vi "FRCts20_Backend_RequestRoot_POST.vi"(6 "Message Attributes":T4, 8 "error in (no error)":errorcluster, 10 "Data":string, 11 "Engine_Refnums":T1) -> (0 "error out":errorcluster)   [LabVIEW 2013, in "FRCts20_Backend_Engine.lvlib"]
doc: "Adds a new request, called by the Request Root API. Expects the team index and description, returns the new request's index"
uses:
  FRCts20_Backend_Engine.lvlib
  Dependencies/Keyed Array/KeyedArray.ctl
  FRCts20_Backend_EngineRefnums.ctl
  INI_Accessor/FRCts20_Backend_INI Controller.lvclass
  Dependencies/AMC/_SubVIs/TypeDefs/Message Queue.ctl
  Dependencies/AMC/_SubVIs/TypeDefs/Message.ctl
  <vilib>/addons/database/Connection.llb/Conn ObjectReference.ctl
  FRCts20_Backend_FGVOperation.ctl
  FRCts20_Backend_API/FRCts20_Backend_API_RequestRoot.ctl
  FRCts20_Backend_API/FRCts20_Backend_API_Status.ctl
  FRCts20_Backend_API/FRCts20_Backend_API.lvlib
  Dependencies/Keyed Array/Tools_KeyedArray.lvlib
  Dependencies/AMC/AMC.lvlib
  <vilib>/addons/database/NI_Database_API.lvlib
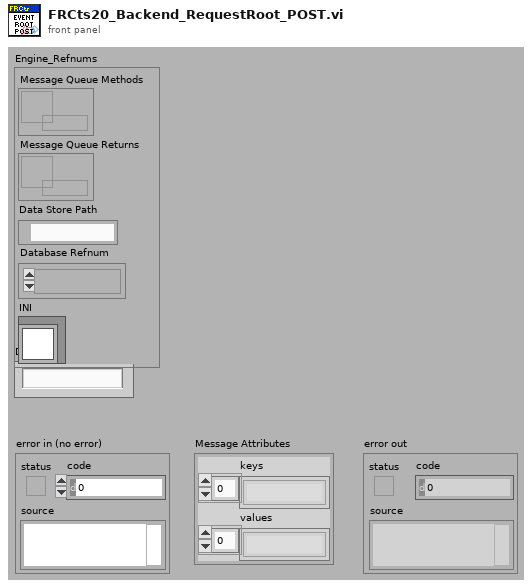
[diagram p1: front panel]
types:
  T1 = typedef "FRCts20_Backend_Engine.lvlib/FRCts20_Backend_EngineRefnums.ctl" = cluster{"Message Queue Methods":T2, "Message Queue Returns":T2, "Data Store Path":path, "Database Refnum":T3, "INI":refnum<class "FRCts20_Backend_INI Controller.lvclass">}
  T2 = typedef "AMC.lvlib/Message Queue.ctl" = refnum<queue>
  T3 = typedef "NI_Database_API.lvlib/Conn ObjectReference.ctl" = refnum<k1>
  T4 = typedef "Tools_KeyedArray.lvlib/KeyedArray.ctl" = cluster{"keys":string[], "values":string[]}
  T5 = typedef "FRCts20_Backend_API.lvlib/FRCts20_Backend_API_RequestRoot.ctl" = cluster{"Requests":cluster{"Request Index":u32, "Description":string, "Status":T6, "Open Date":timestamp, "Last Update":timestamp, "Closed Date":timestamp, "Team Index":u32}[], "APIReturn":string}
  T6 = typedef "FRCts20_Backend_API.lvlib/FRCts20_Backend_API_Status.ctl" = enum16{"Open", "In Work", "Closed"}
  T7 = typedef "FRCts20_Backend_Engine.lvlib/FRCts20_Backend_FGVOperation.ctl" = enum16{"Initialize", "EnqueueMessage", "EnqueueDataReturn", "FlushMessage", "FlushDataReturn"}
  T8 = cluster{"Request Index":u32, "Description":string, "Status":T6, "Open Date":timestamp, "Last Update":timestamp, "Closed Date":timestamp, "Team Index":u32}[]
  T9 = cluster{"Request Index":u32, "Description":string, "Status":T6, "Open Date":timestamp, "Last Update":timestamp, "Closed Date":timestamp, "Team Index":u32}
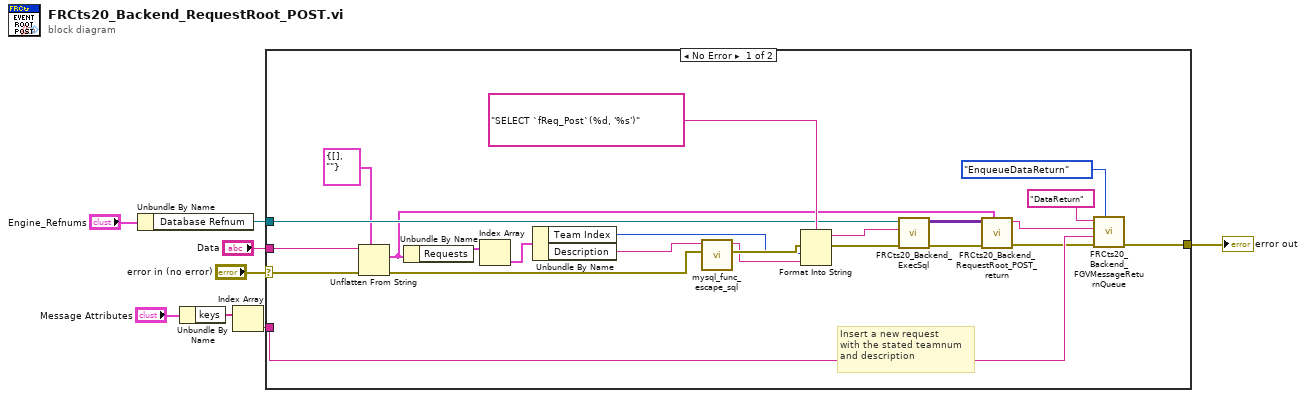
[diagram p0: block diagram]
diagram:
  n1 = Unbundle By Name("Engine_Refnums") -> ("Database Refnum"=w5:T3)
  n2 = Unbundle By Name("Message Attributes") -> ("keys"=w2:string[])
  n3 = Index Array(array=w2) -> (element=w1:string)  [unwired: 1 in]
  n4 = case shown="No Error" "error in (no error)" {
    selector: "error in (no error)" -> [w28 w32]
    tunnel: [w31 w32] -> w7
    tunnel: w5 -> [w21 _]
    tunnel: "Data" -> [w29 _]
    tunnel: w1 -> [w30 _]
    frame No Error {
      # "Insert a new request\nwith the stated teamnum\nand description"
      n5 = Unflatten From String(type=T5 {"Requests"=[], "APIReturn"=""} ("Competition"), binary string=w29, error in (no error)=w28) -> (value=w10:T5, error out=w24:errorcluster)  [unwired: 2 in, 1 out]
      n6 = Unbundle By Name(w10) -> ("Requests"=w15:T8)
      n7 = Index Array(array=w15) -> (element=w14:T9)  [unwired: 1 in]
      n8 = Unbundle By Name(w14) -> ("Team Index"=w12:u32, "Description"=w23:string)
      n9 = call "mysql_func_escape_sql.vi"("error in (no error)"=w24, "sqlin"=w23) -> ("error out"=w22:errorcluster, "escaped"=w11:string)  [unwired: 8 in]
      n10 = Format Into String(format string="SELECT `fReq_Post`(%d, '%s')", error in=w22, w12, w11) -> (resulting string=w20:string, error out=w19:errorcluster)  [unwired: 1 in]
      n11 = call "FRCts20_Backend_ExecSql.vi"("error in (no error)"=w19, "format string"=w20, "Refnum in"=w21) -> ("error out"=w18:errorcluster, "recordset data"=w9:variant[][])  [unwired: 6 in, 1 out]
      n12 = call "FRCts20_Backend_RequestRoot_POST_return.vi"("Request Root"=w10, "error in (no error)"=w18, "recordset data"=w9) -> ("error out"=w17:errorcluster, "data string"=w16:string)  [unwired: 7 in]
      n13 = call "FRCts20_Backend_FGVMessageReturnQueue.vi"("Operation"=FRCts20_Backend_FGVOperation."EnqueueDataReturn", "error in (no error)"=w17, "Key"=w30, "Message Value"=w16, "Message Name"="DataReturn") -> ("error out"=w31:errorcluster)  [unwired: 5 in, 1 out]
    }
    frame Error {
    }
  }
  "error out" <- w7
